vi "FRCts20_Backend_SNS_Publish.vi"(6 "Message Attributes":T1, 8 "error in (no error)":errorcluster, 10 "Data":string, 11 "Engine_Refnums":T2) -> (0 "error out":errorcluster)   [LabVIEW 2014, in "FRCts20_Backend_Engine.lvlib"]
uses:
  FRCts20_Backend_Engine.lvlib
  FRCts20_Backend_EngineRefnums.ctl
  INI_Accessor/FRCts20_Backend_INI Controller.lvclass
  Dependencies/AMC/_SubVIs/TypeDefs/Message Queue.ctl
  Dependencies/AMC/_SubVIs/TypeDefs/Message.ctl
  Dependencies/Keyed Array/KeyedArray.ctl
  <vilib>/addons/database/Connection.llb/Conn ObjectReference.ctl
  FRCts20_Backend_FGVOperation.ctl
  FRCts20_Backend_API/FRCts20_Backend_API_SNS.ctl
  <vilib>/National Instruments/NI Amazon Web Services (AWS) Toolkit for LabVIEW/AWS Core Lib/VI Source/Typedefs/AWS_AWS Credentials.ctl
  <vilib>/National Instruments/NI Amazon Web Services (AWS) Toolkit for LabVIEW/SNS/VI Source/AWS SNS Class/AWS_SNS.lvclass
  <vilib>/National Instruments/NI Amazon Web Services (AWS) Toolkit for LabVIEW/SNS/VI Source/Public Typedefs/AWS_SNS Publish Parameters.ctl
  FRCts20_Backend_API/FRCts20_Backend_API.lvlib
  <vilib>/National Instruments/NI Amazon Web Services (AWS) Toolkit for LabVIEW/SNS/VI Source/AWS_SNS.lvlib
  <vilib>/National Instruments/NI Amazon Web Services (AWS) Toolkit for LabVIEW/AWS Core Lib/VI Source/AWS_Core.lvlib
  Dependencies/Keyed Array/Tools_KeyedArray.lvlib
  Dependencies/AMC/AMC.lvlib
  <vilib>/addons/database/NI_Database_API.lvlib
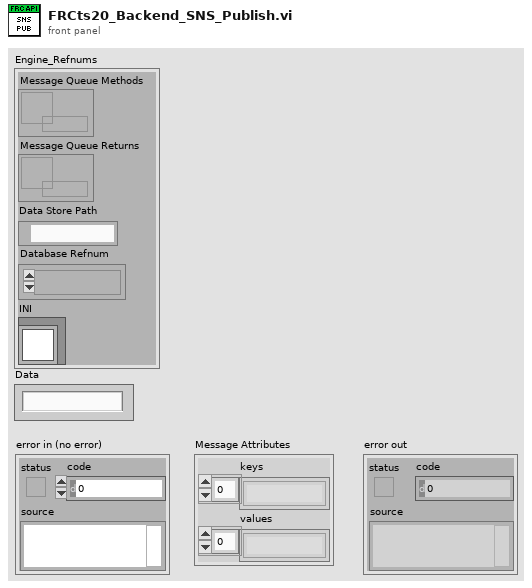
[diagram p1: front panel]
types:
  T1 = typedef "Tools_KeyedArray.lvlib/KeyedArray.ctl" = cluster{"keys":string[], "values":string[]}
  T2 = typedef "FRCts20_Backend_Engine.lvlib/FRCts20_Backend_EngineRefnums.ctl" = cluster{"Message Queue Methods":T3, "Message Queue Returns":T3, "Data Store Path":path, "Database Refnum":T4, "INI":refnum<class "FRCts20_Backend_INI Controller.lvclass">}
  T3 = typedef "AMC.lvlib/Message Queue.ctl" = refnum<queue>
  T4 = typedef "NI_Database_API.lvlib/Conn ObjectReference.ctl" = refnum<k1>
  T5 = typedef "AWS_SNS.lvlib/AWS_SNS Publish Parameters.ctl" = cluster{"Message":string, "Subject":string, "TopicArn":string, "MessageStructure":string}
  T6 = typedef "AWS_Core.lvlib/AWS_AWS Credentials.ctl" = cluster{"AWSAccessKeyId":string, "Secret Key":string}
  T7 = typedef "FRCts20_Backend_API.lvlib/FRCts20_Backend_API_SNS.ctl" = cluster{"Event Name":string, "Team Number":u32, "Subject":string, "Main Message":string, "Phone#":string, "APIReturn":string, "Email":string, "Request Index":u32}
  T8 = typedef "FRCts20_Backend_Engine.lvlib/FRCts20_Backend_FGVOperation.ctl" = enum16{"Initialize", "EnqueueMessage", "EnqueueDataReturn", "FlushMessage", "FlushDataReturn"}
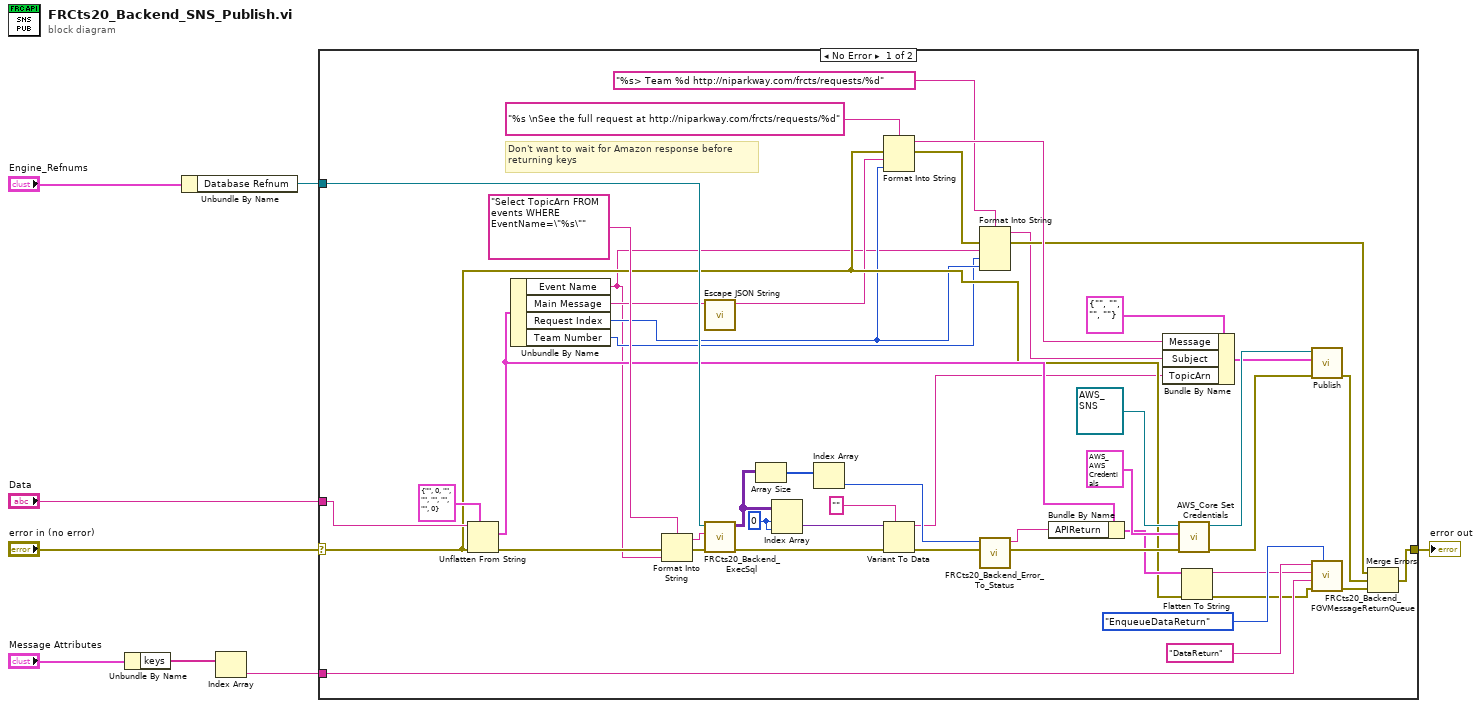
[diagram p0: block diagram]
diagram:
  n1 = Unbundle By Name("Message Attributes") -> ("keys"=w4:string[])
  n2 = Unbundle By Name("Engine_Refnums") -> ("Database Refnum"=w1:T4)
  n3 = Index Array(array=w4) -> (element=w3:string)  [unwired: 1 in]
  n4 = case shown="No Error" "error in (no error)" {
    selector: "error in (no error)" -> [w24 w55]
    tunnel: [w34 w55] -> w7
    tunnel: w1 -> [w43 _]
    tunnel: "Data" -> [w53 _]
    tunnel: w3 -> [w54 _]
    frame No Error {
      w47 = 0 ("index (row)")
      # "Don't want to wait for Amazon response before\nreturning keys"
      n5 = Unflatten From String(type=T7 {"Event Name"="", "Team Number"=0, "Subject"="", "Main Message"="", "Phone#"="", "APIReturn"="", "Email"="", "Request Index"=0} ("SNS"), binary string=w53, error in (no error)=w24) -> (value=w28:T7, error out=w27:errorcluster)  [unwired: 2 in, 1 out]
      n6 = Unbundle By Name(w28) -> ("Event Name"=w9:string, "Main Message"=w32:string, "Request Index"=w11:u32, "Team Number"=w10:u32)
      n7 = Format Into String(format string="Select TopicArn FROM events WHERE EventName=\"%s\"" ("TopicArn"), error in=w27, w9) -> (resulting string=w49:string, error out=w50:errorcluster)  [unwired: 1 in]
      n8 = call "Escape JSON String.vi"("String"=w32) -> ("String Escaped for JSON"=w17:string)  [unwired: 10 in]
      n9 = call "FRCts20_Backend_ExecSql.vi"("error in (no error)"=w50, "format string"=w49, "Refnum in"=w43) -> ("error out"=w51:errorcluster, "recordset data"=w42:variant[][])  [unwired: 6 in, 1 out]
      n10 = Array Size(array=w42) -> (size(s)=w41:i32[])
      n11 = Index Array(array=w42, index (row)=w47, index (col)=w47) -> (element=w46:variant)
      n12 = Index Array(array=w41) -> (element=w40:i32)  [unwired: 1 in]
      n13 = Format Into String(format string="%s \nSee the full request at http://niparkway.com/frcts/requests/%d" ("MessageFormat"), error in=w24, w17, w11) -> (resulting string=w22:string, error out=w16:errorcluster)  [unwired: 1 in]
      n14 = Variant To Data(error in=w51, type="" ("TopicArn"), Variant=w46) -> (data=w19:string, error out=w39:errorcluster)
      n15 = Format Into String(format string="%s> Team %d http://niparkway.com/frcts/requests/%d" ("Subject"), error in=w16, w9, w10, w11) -> (resulting string=w12:string, error out=w15:errorcluster)  [unwired: 1 in]
      n16 = call "FRCts20_Backend_Error_To_Status.vi"("error in (no error)"=w39, "rows affected"=w40) -> ("error out"=w36:errorcluster, "String"=w29:string)  [unwired: 8 in]
      n17 = Bundle By Name(cluster=w28, "APIReturn"=w29) -> (w26:T7)
      n18 = Bundle By Name(cluster=T5 {"Message"="", "Subject"="", "TopicArn"="", "MessageStructure"=""} ("Publish Parameters"), "Message"=w22, "Subject"=w12, "TopicArn"=w19) -> (w21:T5)
      n19 = call-dynamic "AWS_Core Set Credentials.vi"("error in (no error)"=w36, "AWS Credentials"=T6 {"AWSAccessKeyId"="AKIAIBWID7GQA3ZVLBGQ", "Secret Key"="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"}, "AWS_Core in"=refnum<class "AWS_SNS.lvclass"> refnum ("AWS_SNS in")) -> ("error out"=w37:errorcluster, "AWS_Core out"=w38:refnum<class "AWS_SNS.lvclass">)  [unwired: 7 in]
      n20 = Flatten To String(anything=w26, error in (no error)=w24) -> (data string=w25:string, error out=w23:errorcluster)  [unwired: 2 in, 1 out]
      n21 = call-dynamic "Publish.vi"("AWS_SNS in"=w38, "Publish Parameters"=w21, "error in (no error)"=w37) -> ("error out"=w14:errorcluster)  [unwired: 5 in, 2 out]
      n22 = call "FRCts20_Backend_FGVMessageReturnQueue.vi"("Operation"=FRCts20_Backend_FGVOperation."EnqueueDataReturn", "error in (no error)"=w23, "Key"=w54, "Message Value"=w25, "Message Name"="DataReturn") -> ("error out"=w35:errorcluster)  [unwired: 5 in, 1 out]
      n23 = Merge Errors(w15, w14, w35) -> (w34:errorcluster)
    }
    frame Error {
    }
  }
  "error out" <- w7
